vi "main.vi"() -> (1 "RMD":T3, 2 "RQD":T3={"Y20 2"=FALSE, "Y21 2"=FALSE, "Y22 2"=FALSE, "Y24 2"=FALSE, "Y23 2"=FALSE, "Y25 2"=FALSE, "Y26 2"=FALSE, "Y27 2"=FALSE, "Y10 2"=FALSE, "Y11 2"=FALSE, "Y12 2"=FALSE, "Y13 2"=FALSE, "Y14 2"=FALSE, "Y15 2"=FALSE, "Y16 2"=FALSE, "Y17 2"=FALSE, "Y0 2"=TRUE, "Y1 2"=TRUE, "Y2 2"=TRUE, "Y3 2"=TRUE, "Y4 2"=TRUE, "Y5 2"=FALSE, "Y6 2"=FALSE, "Y7 2"=FALSE, "Y30 2"=FALSE, "Y31 2"=FALSE, "Y32 2"=FALSE, "Y33 2"=FALSE, "Y34  2"=FALSE, "Y35  2"=FALSE, "Y36 2"=FALSE, "Y37 2"=FALSE}, 3 "RID":T5)   [LabVIEW 2014]
panel:
  in  "M点输入":bool[](array[boolean])
  in  "VW输入":i16[](array[numeric])
  out "VW区":i16[](array[numeric])
  out "M点读取":bool[](array[boolean])
  in  "VD":T1
  in  "PLC 系列":u8(ring) items=["1200.200.200SMART"=0, "S7-300"=2, "S7-400"=3]
  in  "VW":T2={"VW0"=30, "VW2"=0, "VW4"=0, "VW6"=0, "VW8"=0, "VW10"=0, "VW12"=0, "VW14"=0, "VW16"=0, "VW18"=0, "VW20"=0, "VW22"=0, "VW24"=0, "VW26"=0, "VW28"=0, "VW30"=0, "VW32"=0, "VW34"=0, "VW36"=0, "VW38"=0, "VW40"=0, "VW42"=0, "VW44"=0, "VW46"=0}
  in  "WMD":T4
  in  "WQD":T4
  in  "停止":bool
  # "MX.0"
  # "QX.0-QX.7"
  # "IX.0-IX.7"
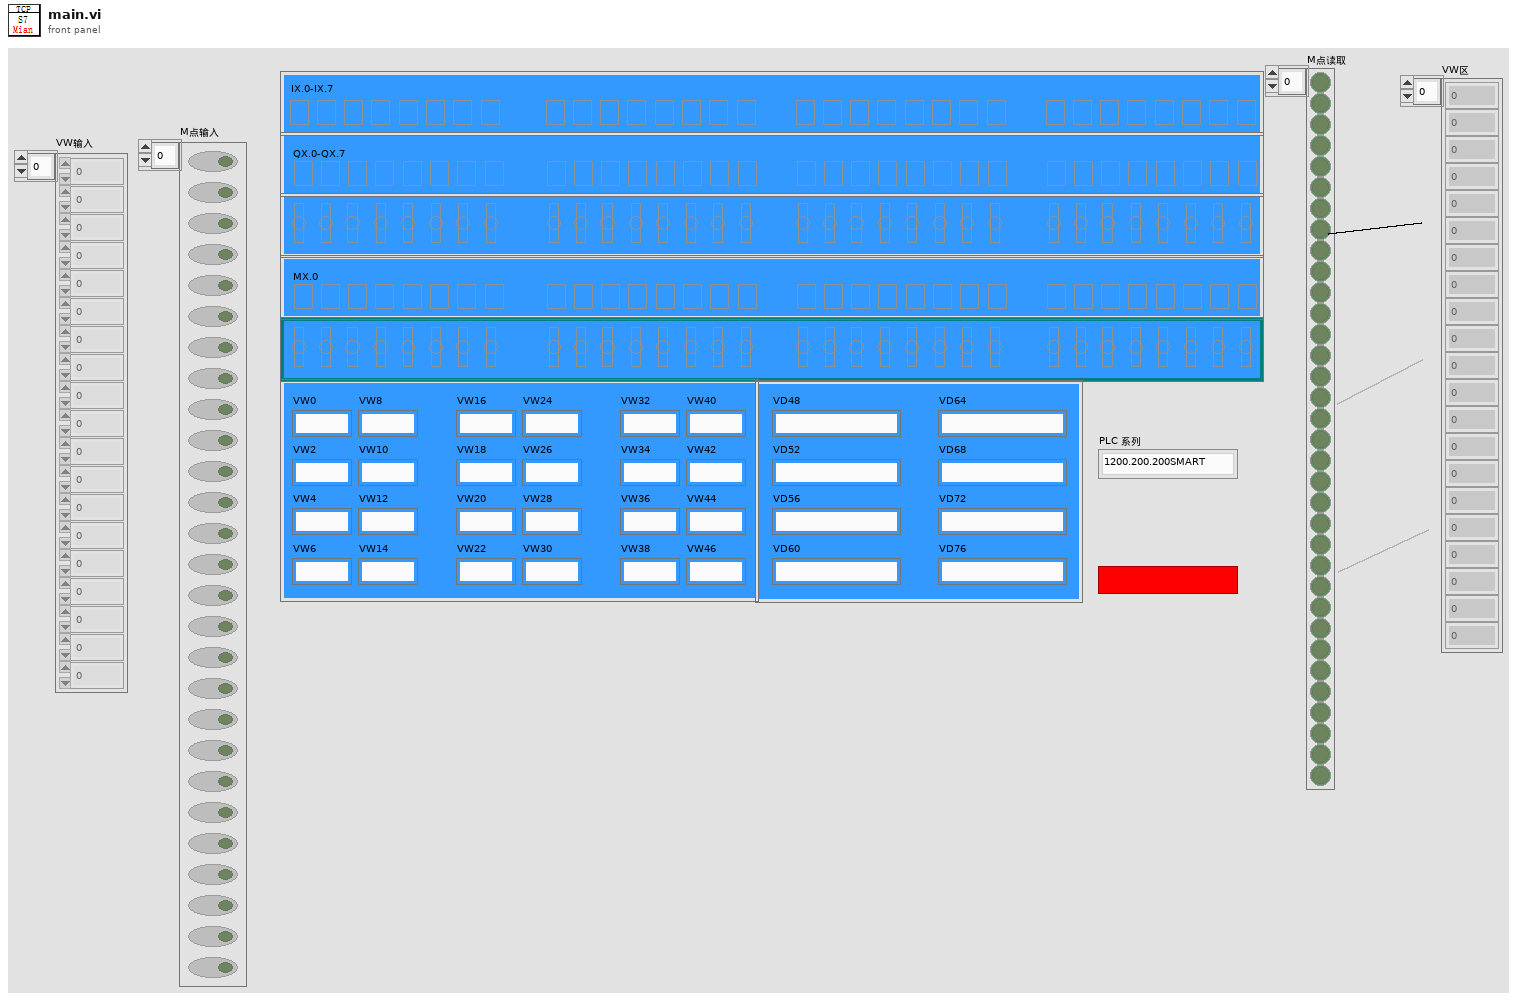
[diagram p1: front panel]
types:
  T1 = cluster{"VD48":u32, "VD52":u32, "VD56":u32, "VD60":u32, "VD64":u32, "VD68":u32, "VD72":u32, "VD76":u32}
  T2 = cluster{"VW0":u16, "VW2":u16, "VW4":u16, "VW6":u16, "VW8":u16, "VW10":u16, "VW12":u16, "VW14":u16, "VW16":u16, "VW18":u16, "VW20":u16, "VW22":u16, "VW24":u16, "VW26":u16, "VW28":u16, "VW30":u16, "VW32":u16, "VW34":u16, "VW36":u16, "VW38":u16, "VW40":u16, "VW42":u16, "VW44":u16, "VW46":u16}
  T3 = cluster{"Y20 2":bool, "Y21 2":bool, "Y22 2":bool, "Y24 2":bool, "Y23 2":bool, "Y25 2":bool, "Y26 2":bool, "Y27 2":bool, "Y10 2":bool, "Y11 2":bool, "Y12 2":bool, "Y13 2":bool, "Y14 2":bool, "Y15 2":bool, "Y16 2":bool, "Y17 2":bool, "Y0 2":bool, "Y1 2":bool, "Y2 2":bool, "Y3 2":bool, "Y4 2":bool, "Y5 2":bool, "Y6 2":bool, "Y7 2":bool, "Y30 2":bool, "Y31 2":bool, "Y32 2":bool, "Y33 2":bool, "Y34  2":bool, "Y35  2":bool, "Y36 2":bool, "Y37 2":bool}
  T4 = cluster{"Q3.0":bool, "Q3.1":bool, "Q3.2":bool, "Q3.3":bool, "Q3.4":bool, "Q3.5":bool, "Q3.6":bool, "Q3.7":bool, "Q2.0":bool, "Q2.1":bool, "Q2.2":bool, "Q2.3":bool, "Q2.4":bool, "Q2.5":bool, "Q2.6":bool, "Q2.7":bool, "Q1.0":bool, "Q1.1":bool, "Q1.2":bool, "Q1.3":bool, "Q1.4":bool, "Q1.5":bool, "Q1.6":bool, "Q1.7":bool, "Q0.0":bool, "Q0.1":bool, "Q0.2":bool, "Q0.3":bool, "Q0.4":bool, "Q0.5":bool, "Q0.6":bool, "Q0.7":bool}
  T5 = cluster{"X20":bool, "X21":bool, "X22":bool, "X24":bool, "X23":bool, "X25":bool, "X26":bool, "X27":bool, "X10":bool, "X11":bool, "X12":bool, "X13":bool, "X14":bool, "X15":bool, "X16":bool, " X17":bool, "X0":bool, "X1":bool, "X2":bool, "X3":bool, "X4":bool, "X5":bool, "X6":bool, "X7":bool, "X30":bool, "X31":bool, "X32":bool, "X33":bool, "X34 ":bool, "X35 ":bool, "X36":bool, "X37":bool}
  T6 = typedef "运行步骤控件.ctl" = enum16{"RI", "RQ", "RM", "RV"}
  T7 = cluster{"Boolean array[0]":bool, "Boolean array[1]":bool, "Boolean array[2]":bool, "Boolean array[3]":bool, "Boolean array[4]":bool, "Boolean array[5]":bool, "Boolean array[6]":bool, "Boolean array[7]":bool, "Boolean array[8]":bool, "Boolean array[9]":bool, "Boolean array[10]":bool, "Boolean array[11]":bool, "Boolean array[12]":bool, "Boolean array[13]":bool, "Boolean array[14]":bool, "Boolean array[15]":bool, "Boolean array[16]":bool, "Boolean array[17]":bool, "Boolean array[18]":bool, "Boolean array[19]":bool, "Boolean array[20]":bool, "Boolean array[21]":bool, "Boolean array[22]":bool, "Boolean array[23]":bool, "Boolean array[24]":bool, "Boolean array[25]":bool, "Boolean array[26]":bool, "Boolean array[27]":bool, "Boolean array[28]":bool, "Boolean array[29]":bool, "Boolean array[30]":bool, "Boolean array[31]":bool}
  T8 = cluster{"[0]":u32, "[1]":u32, "[2]":u32, "[3]":u32, "[4]":u32, "[5]":u32, "[6]":u32, "[7]":u32}
  T9 = cluster{"[0]":u16, "[1]":u16, "[2]":u16, "[3]":u16, "[4]":u16, "[5]":u16, "[6]":u16, "[7]":u16, "[8]":u16, "[9]":u16, "[10]":u16, "[11]":u16, "[12]":u16, "[13]":u16, "[14]":u16, "[15]":u16, "[16]":u16, "[17]":u16, "[18]":u16, "[19]":u16, "[20]":u16, "[21]":u16, "[22]":u16, "[23]":u16}
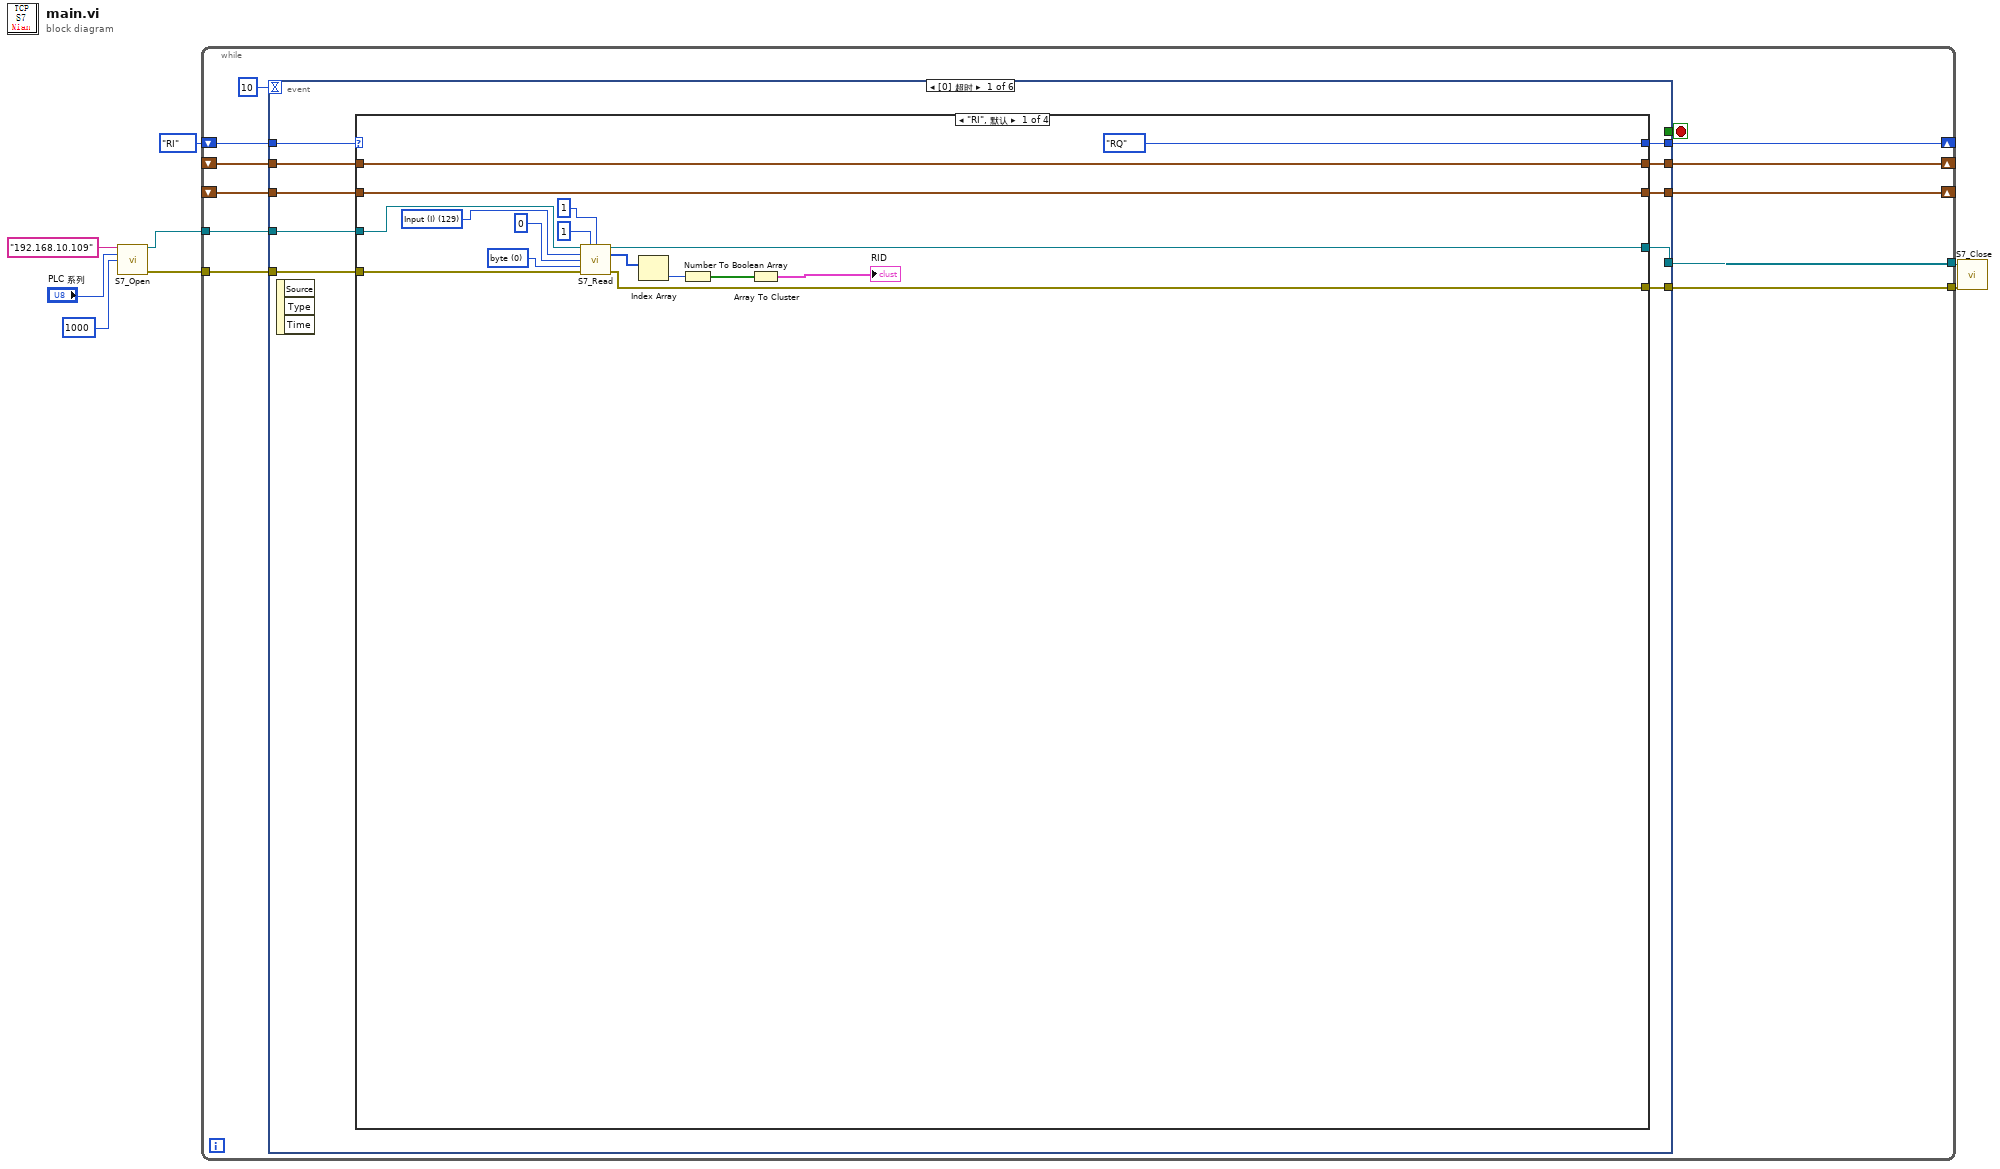
[diagram p0: block diagram]
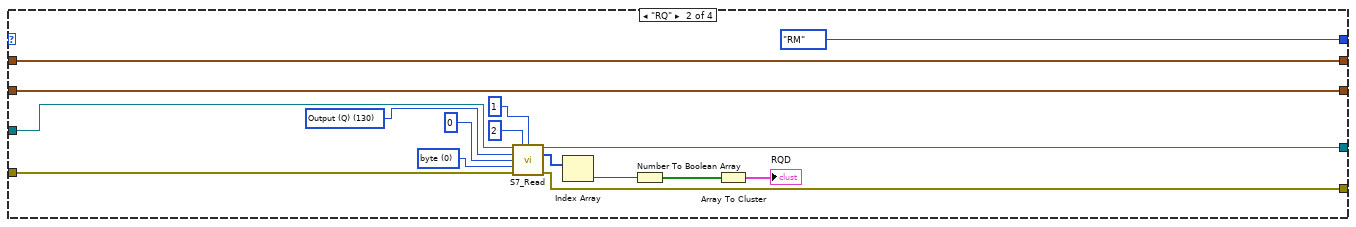
[diagram p2: hidden frame]
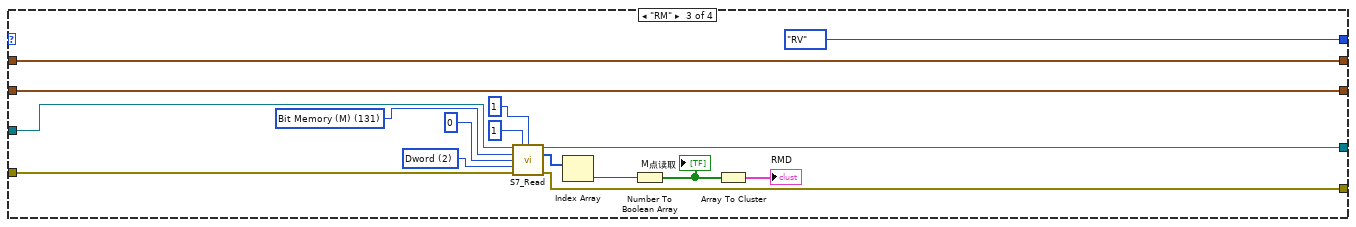
[diagram p3: hidden frame]
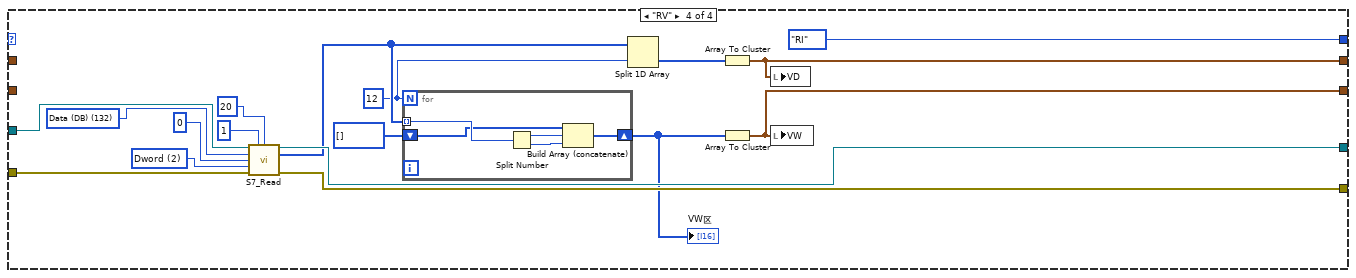
[diagram p4: hidden frame]
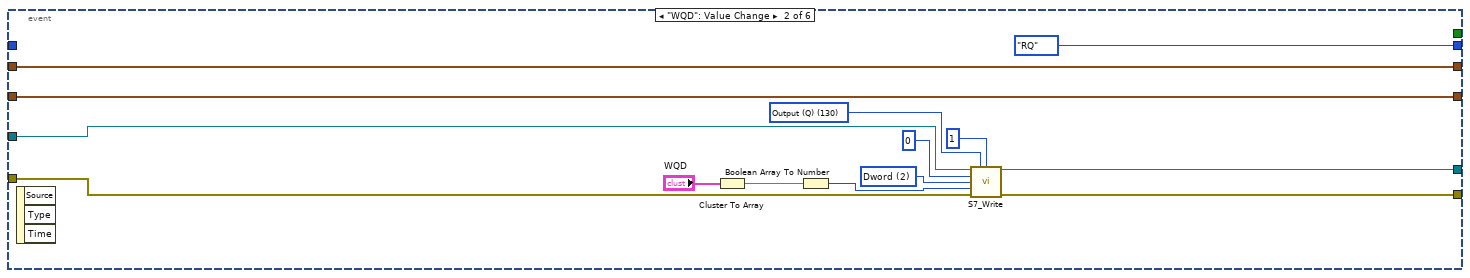
[diagram p5: hidden frame]
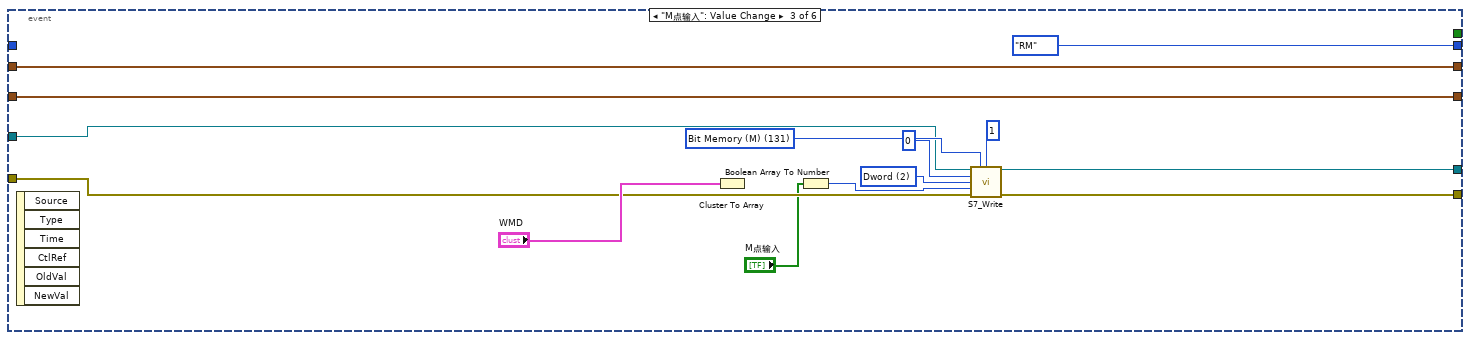
[diagram p6: hidden frame]
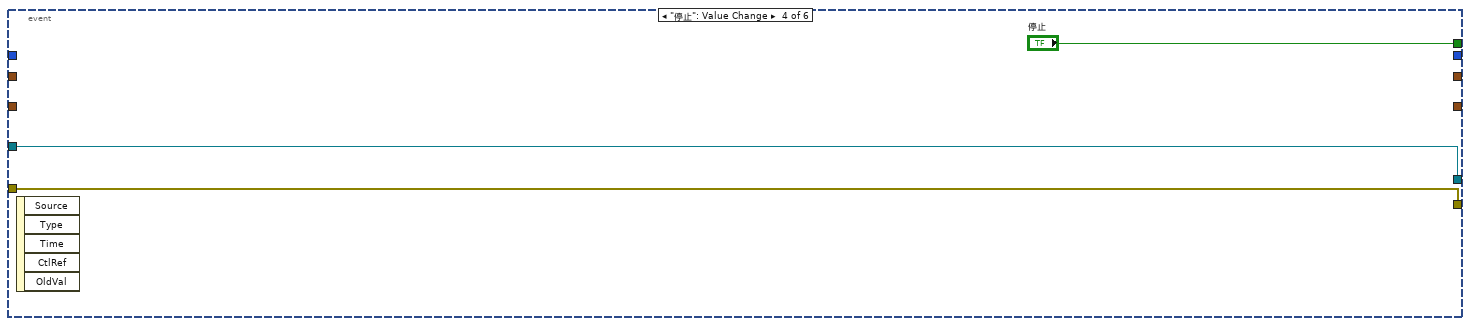
[diagram p7: hidden frame]
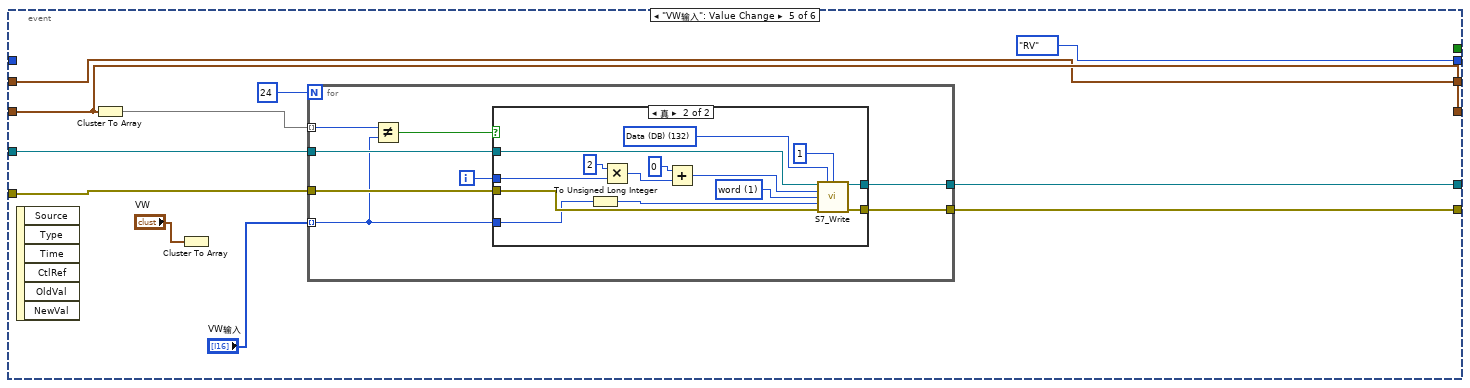
[diagram p8: hidden frame]
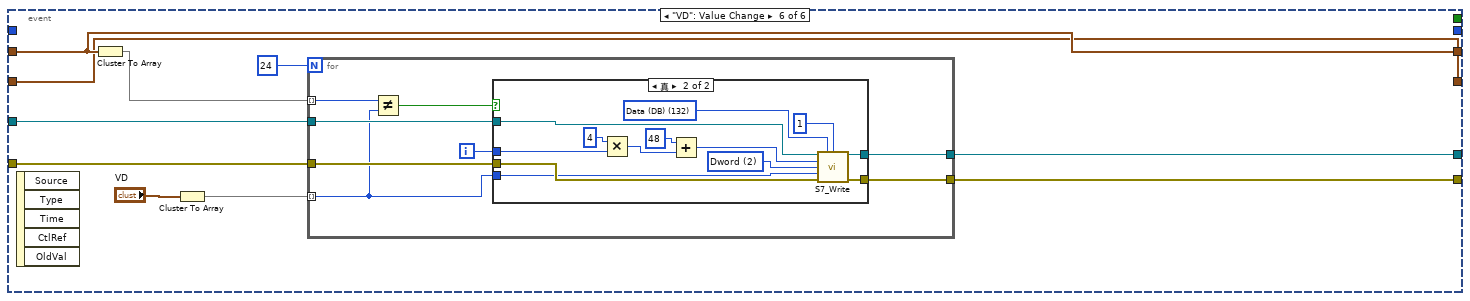
[diagram p10: hidden frame]
diagram:
  n1 = call "S7_Open.vi"("IP 地址"="192.168.10.109", "PLC 系列"="PLC 系列", "超时（MS）"=1000) -> ("TCP"=w7:refnum<k5>, "error out"=w6:errorcluster)  [unwired: 2 in, 9 out]
  n2 = while {
    tunnel: w7 -> [w19]
    tunnel: w6 -> [w18]
    tunnel: [w17] -> w5
    tunnel: [w16] -> w4
    shift-right: [w14] -> _
    shift-left: 运行步骤控件."RI" ("枚举") -> [w15]
    shift-right: [w13] -> _
    shift-left: _ -> [w11]
    shift-right: [w12] -> _
    shift-left: _ -> [w10]
    stop <- w9 stop-if-true
    n3 = event shown="[0] 超时" {
      selector: _ -> [_ _ _ _ _ _]
      dyn-events: _ -> [_ _ _ _ _ _]
      timeout: 10 -> [_ _ _ _ _ _]
      tunnel: w19 -> [w30 w114 w121 w130 w140 w172]
      tunnel: w18 -> [w29 w113 w119 w129 w139 w171]
      tunnel: [w28 w112 w123 w130 w142 w170] -> w17
      tunnel: [w27 w111 w122 w129 w141 w169] -> w16
      tunnel: w15 -> [w26 _ _ _ _ _]
      tunnel: [w25 运行步骤控件."RQ" ("枚举") 运行步骤控件."RM" ("枚举") _ 运行步骤控件."RV" ("枚举") _] -> w14
      tunnel: [w24 w103 w118 _ w135 w167] -> w13
      tunnel: [w23 w102 w117 _ w134 w168] -> w12
      tunnel: w11 -> [w22 w103 w118 _ w135 w167]
      tunnel: w10 -> [w21 w102 w117 _ w134 w168]
      tunnel: [_ _ _ "停止" _ _] -> w9
      event Timeout {
        n4 = event-data() -> ()  [unwired: 4 out]
        n5 = case shown="\"RI\", 默认" w26 {
          tunnel: w30 -> [w42 w62 w70 w88]
          tunnel: w29 -> [w37 w61 w69 w87]
          tunnel: [w41 w60 w72 w90] -> w28
          tunnel: [w40 w59 w71 w89] -> w27
          tunnel: [运行步骤控件."RQ" ("枚举") 运行步骤控件."RM" ("枚举") 运行步骤控件."RV" ("枚举") 运行步骤控件."RI" ("枚举")] -> w25
          tunnel: [w32 w50 w64 w81] -> w24
          tunnel: [w31 w49 w63 w80] -> w23
          tunnel: w22 -> [w32 w50 w64 _]
          tunnel: w21 -> [w31 w49 w63 _]
          frame "RI", Default {
            w43 = u16 0 items=["byte", "word", "Dword"] ("数据类型")
            w39 = u8 129 items=["I/O (P)"=128, "Input (I)"=129, "Output (Q)"=130, "Bit Memory (M)"=131, "Data (DB)"=132, "Instance Data (DI)"=133, "Local Data (L)"=134, "Predecessor Local Data (VL)"=135] ("寄存器类型")
            n6 = call "S7_Read.vi"("TCP"=w42, "DB #"=u16 1, "读取长度"=u16 1, "寄存器类型"=w39, "起始地址"=u32 0, "数据类型"=w43, "error in"=w37) -> ("TCP"=w41:refnum<k5>, "数据"=w35:u32[], "error out"=w40:errorcluster)  [unwired: 6 out]
            n7 = Index Array(array=w35) -> (element=w34:u32)  [unwired: 1 in]
            n8 = Number To Boolean Array(number=w34) -> (Boolean array=w33:bool[])
            n9 = Array To Cluster(array=w33) -> (cluster=→"RID":T7)
          }
          frame "RQ" {
            w54 = u16 0 items=["byte", "word", "Dword"] ("数据类型")
            w56 = u8 130 items=["I/O (P)"=128, "Input (I)"=129, "Output (Q)"=130, "Bit Memory (M)"=131, "Data (DB)"=132, "Instance Data (DI)"=133, "Local Data (L)"=134, "Predecessor Local Data (VL)"=135] ("寄存器类型")
            n10 = call "S7_Read.vi"("TCP"=w62, "DB #"=u16 2, "读取长度"=u16 1, "寄存器类型"=w56, "起始地址"=u32 0, "数据类型"=w54, "error in"=w61) -> ("TCP"=w60:refnum<k5>, "数据"=w52:u32[], "error out"=w59:errorcluster)  [unwired: 6 out]
            n11 = Index Array(array=w52) -> (element=w51:u32)  [unwired: 1 in]
            n12 = Number To Boolean Array(number=w51) -> (Boolean array=w48:bool[])
            n13 = Array To Cluster(array=w48) -> (cluster=→"RQD":T7)
          }
          frame "RM" {
            w73 = u16 2 items=["byte", "word", "Dword"] ("数据类型")
            w77 = u8 131 items=["I/O (P)"=128, "Input (I)"=129, "Output (Q)"=130, "Bit Memory (M)"=131, "Data (DB)"=132, "Instance Data (DI)"=133, "Local Data (L)"=134, "Predecessor Local Data (VL)"=135] ("寄存器类型")
            n14 = call "S7_Read.vi"("TCP"=w70, "DB #"=u16 1, "读取长度"=u16 1, "寄存器类型"=w77, "起始地址"=u32 0, "数据类型"=w73, "error in"=w69) -> ("TCP"=w72:refnum<k5>, "数据"=w66:u32[], "error out"=w71:errorcluster)  [unwired: 6 out]
            n15 = Index Array(array=w66) -> (element=w68:u32)  [unwired: 1 in]
            n16 = Number To Boolean Array(number=w68) -> (Boolean array=w67:bool[])
            "M点读取" <- w67
            n17 = Array To Cluster(array=w67) -> (cluster=→"RMD":T7)
          }
          frame "RV" {
            w91 = u16 2 items=["byte", "word", "Dword"] ("数据类型")
            w95 = u8 132 items=["I/O (P)"=128, "Input (I)"=129, "Output (Q)"=130, "Bit Memory (M)"=131, "Data (DB)"=132, "Instance Data (DI)"=133, "Local Data (L)"=134, "Predecessor Local Data (VL)"=135] ("寄存器类型")
            w79 = 12
            n18 = call "S7_Read.vi"("TCP"=w88, "DB #"=u16 1, "读取长度"=u16 20, "寄存器类型"=w95, "起始地址"=u32 0, "数据类型"=w91, "error in"=w87) -> ("TCP"=w90:refnum<k5>, "数据"=w84:u32[], "error out"=w89:errorcluster)  [unwired: 6 out]
            n19 = for {
              N: w79 -> [_]
              tunnel: w84 -> [w100] mode=indexing
              shift-right: [w99] -> w83
              shift-left: u16[] [] -> [w98]
              n20 = Split Number(x=w100) -> (hi(x)=w97:u16, lo(x)=w96:u16)
              n21 = Build Array (concatenate)(w98, w97, w96) -> (w99:u16[])
            }
            "VW区" <- w83
            n22 = Split 1D Array(array=w84, index=w79) -> (second subarray=w82:u32[])  [unwired: 1 out]
            n23 = Array To Cluster(array=w82) -> (cluster=w80:T8)
            n24 = Array To Cluster(array=w83) -> (cluster=w81:T9)
            n25 = local write "VD"(w80) -> ()
            n26 = local write "VW"(w81) -> ()
          }
        }
      }
      event "WQD": Value Change {
        w107 = u16 2 items=["byte", "word", "Dword"] ("数据类型")
        w110 = u8 130 items=["I/O (P)"=128, "Input (I)"=129, "Output (Q)"=130, "Bit Memory (M)"=131, "Data (DB)"=132, "Instance Data (DI)"=133, "Local Data (L)"=134, "Predecessor Local Data (VL)"=135] ("寄存器类型")
        n27 = event-data() -> ()  [unwired: 4 out]
        n28 = Cluster To Array(cluster="WQD") -> (array=w105:bool[])
        n29 = Boolean Array To Number(Boolean array=w105) -> (number=w104:u32)
        n30 = call "S7_Write.vi"("TCP"=w114, "寄存器类型"=w110, "DB #"=u16 1, "写入地址"=u32 0, "数据类型"=w107, "写入数据"=w104, "error in"=w113) -> ("TCP"=w112:refnum<k5>, "error out"=w111:errorcluster)  [unwired: 7 out]
      }
      event "M点输入": Value Change {
        w125 = u16 2 items=["byte", "word", "Dword"] ("数据类型")
        w128 = u8 131 items=["I/O (P)"=128, "Input (I)"=129, "Output (Q)"=130, "Bit Memory (M)"=131, "Data (DB)"=132, "Instance Data (DI)"=133, "Local Data (L)"=134, "Predecessor Local Data (VL)"=135] ("寄存器类型")
        n31 = event-data() -> ()  [unwired: 7 out]
        n32 = Cluster To Array(cluster="WMD") -> ()  [unwired: 1 out]
        n33 = Boolean Array To Number(Boolean array="M点输入") -> (number=w124:u32)
        n34 = call "S7_Write.vi"("TCP"=w121, "寄存器类型"=w128, "DB #"=u16 1, "写入地址"=u32 0, "数据类型"=w125, "写入数据"=w124, "error in"=w119) -> ("TCP"=w123:refnum<k5>, "error out"=w122:errorcluster)  [unwired: 7 out]
      }
      event "停止": Value Change {
        n35 = event-data() -> ()  [unwired: 6 out]
      }
      event "VW输入": Value Change {
        n36 = event-data() -> ()  [unwired: 7 out]
        n37 = Cluster To Array(cluster=w135) -> (array=w136:u16[])
        n38 = Cluster To Array(cluster="VW") -> ()  [unwired: 1 out]
        n39 = for {
          N: 24 -> [_]
          tunnel: [w150] -> w142
          tunnel: [w149] -> w141
          tunnel: w140 -> [w148]
          tunnel: w139 -> [w147]
          tunnel: w136 -> [w146] mode=indexing
          tunnel: "VW输入" -> [w144] mode=indexing
          i -> [w143]
          n40 = Not Equal?(x=w146, y=w144) -> (x != y?=w145:bool)
          n41 = case shown="真" w145 {
            tunnel: [w152 w163] -> w150
            tunnel: [w151 w162] -> w149
            tunnel: w148 -> [w152 w161]
            tunnel: w147 -> [w151 w160]
            tunnel: w144 -> [_ w155]
            tunnel: w143 -> [_ w157]
            frame False {
            }
            frame True {
              w164 = u16 1 items=["byte", "word", "Dword"] ("数据类型")
              w166 = u8 132 items=["I/O (P)"=128, "Input (I)"=129, "Output (Q)"=130, "Bit Memory (M)"=131, "Data (DB)"=132, "Instance Data (DI)"=133, "Local Data (L)"=134, "Predecessor Local Data (VL)"=135] ("寄存器类型")
              n42 = To Unsigned Long Integer(number=w155) -> (unsigned 32bit integer=w154:u32)
              n43 = Multiply(x=u32 2, y=w157) -> (x*y=w158:u32)
              n44 = Add(x=u32 0 ("写入地址"), y=w158) -> (x+y=w153:u32)
              n45 = call "S7_Write.vi"("TCP"=w161, "寄存器类型"=w166, "DB #"=u16 1, "写入地址"=w153, "数据类型"=w164, "写入数据"=w154, "error in"=w160) -> ("TCP"=w163:refnum<k5>, "error out"=w162:errorcluster)  [unwired: 7 out]
            }
          }
        }
      }
      event "VD": Value Change {
        n46 = event-data() -> ()  [unwired: 6 out]
        n47 = Cluster To Array(cluster=w168) -> (array=w175:u32[])
        n48 = Cluster To Array(cluster="VD") -> (array=w174:u32[])
        n49 = for {
          N: 24 -> [_]
          tunnel: [w184] -> w170
          tunnel: [w183] -> w169
          tunnel: w172 -> [w182]
          tunnel: w171 -> [w181]
          tunnel: w175 -> [w180] mode=indexing
          tunnel: w174 -> [w178] mode=indexing
          i -> [w177]
          n50 = Not Equal?(x=w180, y=w178) -> (x != y?=w179:bool)
          n51 = case shown="真" w179 {
            tunnel: [w186 w196] -> w184
            tunnel: [w185 w195] -> w183
            tunnel: w182 -> [w186 w194]
            tunnel: w181 -> [w185 w193]
            tunnel: w178 -> [_ w187]
            tunnel: w177 -> [_ w190]
            frame False {
            }
            frame True {
              w197 = u16 2 items=["byte", "word", "Dword"] ("数据类型")
              w199 = u8 132 items=["I/O (P)"=128, "Input (I)"=129, "Output (Q)"=130, "Bit Memory (M)"=131, "Data (DB)"=132, "Instance Data (DI)"=133, "Local Data (L)"=134, "Predecessor Local Data (VL)"=135] ("寄存器类型")
              n52 = Multiply(x=u32 4, y=w190) -> (x*y=w191:u32)
              n53 = Add(x=u32 48 ("写入地址"), y=w191) -> (x+y=w188:u32)
              n54 = call "S7_Write.vi"("TCP"=w194, "寄存器类型"=w199, "DB #"=u16 1, "写入地址"=w188, "数据类型"=w197, "写入数据"=w187, "error in"=w193) -> ("TCP"=w196:refnum<k5>, "error out"=w195:errorcluster)  [unwired: 7 out]
            }
          }
        }
      }
    }
  }
  n55 = call "S7_Close.vi"("error in"=w4, "TCP Connection Ref"=w5) -> ()  [unwired: 10 out]
